vi "cam create grab.vi"(8 "error in (no error)":errorcluster, 10 "Resolution Selection":u16, 11 "Refnum in":T1) -> (0 "error out":errorcluster, 1 "Width":u32, 2 "Height":u32, 3 "Refnum out":T1)   [LabVIEW 2024]
uses:
  <vilib>/userDefined/High Color/IMAQdx.ctl
  <resource>/objmgr/imaqdx.rc
  <vilib>/vision/driver/NI_Vision_Acquisition_Software.lvlib
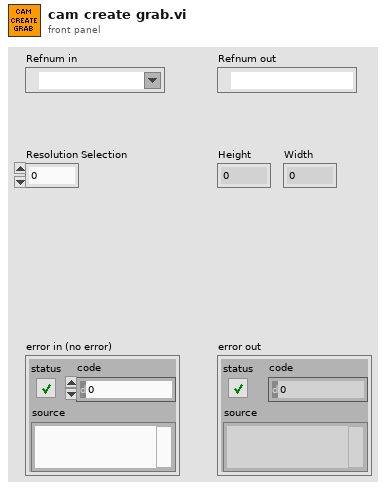
[diagram p1: front panel]
types:
  T1 = typedef "IMAQdx.ctl" = refnum<k21>
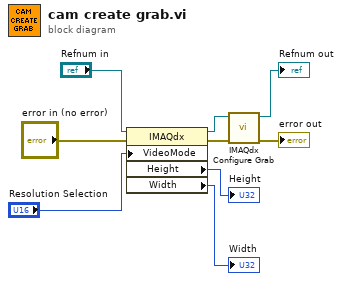
[diagram p0: block diagram]
diagram:
  n1 = property class="IMAQdx"(reference="Refnum in", error in="error in (no error)", "VideoMode"="Resolution Selection") -> (reference out=w7:T1, error out=w6:errorcluster, "Height"=→"Height":u32, "Width"=→"Width":u32)
  n2 = call <vilib>:"IMAQdx Configure Grab.vi"("error in"=w6, "Session In"=w7) -> ("error out"=→"error out":errorcluster, "Session Out"=→"Refnum out":T1)  [unwired: 8 in]
